vi "Find Next Available DigPatrn FPGA Resource and Name.vi"(9 "FPGA Resources":string[](array[string]), 10 "Patterns":T1[](array[typedef]), 11 "New Pattern in":T1) -> (3 "New Pattern out":T1)   [LabVIEW 2015, in "Engine Simulation Toolkit System Explorer.lvlib"]
uses:
  Engine Simulation Toolkit System Explorer.lvlib
  Digital Pattern.ctl
  Digital Pattern Base.ctl
  Digital Pattern Remove Edge.ctl
  Digital Pattern Add Pulse.ctl
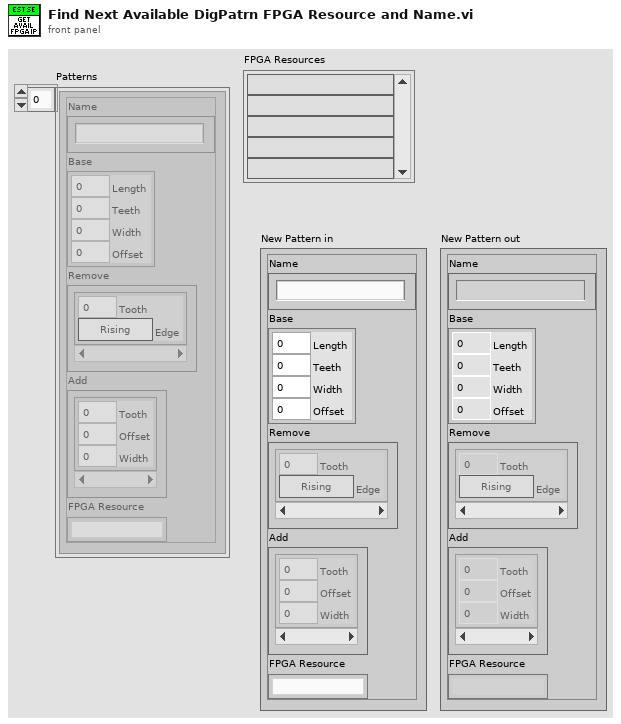
[diagram p1: front panel]
types:
  T1 = typedef "Engine Simulation Toolkit System Explorer.lvlib/Digital Pattern.ctl" = cluster{"Name":string, "Base":T2, "Remove":T3[], "Add":T4[], "FPGA Resource":string}
  T2 = typedef "Engine Simulation Toolkit System Explorer.lvlib/Digital Pattern Base.ctl" = cluster{"Length":dbl, "Teeth":u16, "Width":dbl, "Offset":dbl}
  T3 = typedef "Engine Simulation Toolkit System Explorer.lvlib/Digital Pattern Remove Edge.ctl" = cluster{"Tooth":u16, "Edge":bool}
  T4 = typedef "Engine Simulation Toolkit System Explorer.lvlib/Digital Pattern Add Pulse.ctl" = cluster{"Tooth":u16, "Offset":dbl, "Width":dbl}
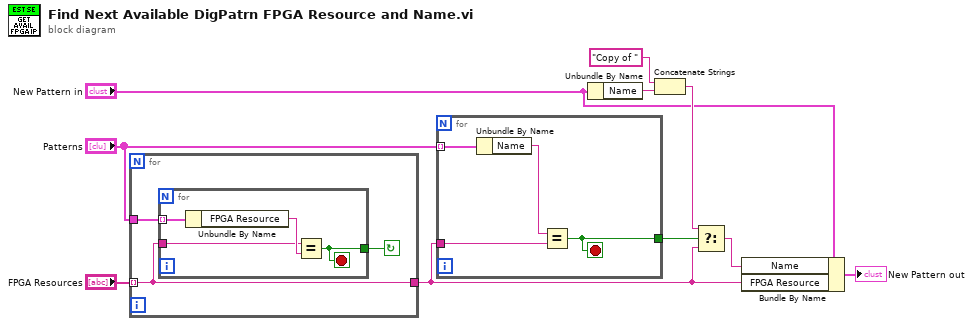
[diagram p0: block diagram]
diagram:
  n1 = for {
    tunnel: "FPGA Resources" -> [w12] mode=indexing
    tunnel: "Patterns" -> [w13]
    tunnel: [w12] -> w2
    stop <- w11 continue-if-true
    n2 = for {
      tunnel: w13 -> [w17] mode=indexing
      tunnel: w12 -> [w15]
      tunnel: [w14] -> w11
      stop <- w14 stop-if-true
      n3 = Unbundle By Name(w17) -> ("FPGA Resource"=w16:string)
      n4 = Equal?(x=w15, y=w16) -> (x = y?=w14:bool)
    }
  }
  n5 = for {
    tunnel: "Patterns" -> [w20] mode=indexing
    tunnel: w2 -> [w21]
    tunnel: [w18] -> w8
    stop <- w18 stop-if-true
    n6 = Unbundle By Name(w20) -> ("Name"=w19:string)
    n7 = Equal?(x=w19, y=w21) -> (x = y?=w18:bool)
  }
  n8 = Unbundle By Name("New Pattern in") -> ("Name"=w5:string)
  n9 = Concatenate Strings("Copy of " ("string"), w5) -> (w6:string)
  n10 = Select(t=w6, s=w8, f=w2) -> (s? t:f=w3:string)
  n11 = Bundle By Name(cluster="New Pattern in", "Name"=w3, "FPGA Resource"=w2) -> (→"New Pattern out":T1)
